vi "Set Combobox Font.vi"(6 "Combo Box Ref":refnum<vi>, 8 "error in (no error)":errorcluster, 9 "Font Size (0: No Change)":i32, 10 "Font (\"\": No Change)":string, 11 "Path Selector in":refnum<class "MGI Path Selector.lvclass">) -> (0 "error out":errorcluster, 3 "Path Selector out":refnum<class "MGI Path Selector.lvclass">)   [LabVIEW 2020, in "MGI Path Selector.lvclass"]
doc: "Update the specified combo box's font and size as specified.\n\nAuthored by Shawn Walpole\nsupport@mooregoodideas.com\nwww.mooregoodideas.com\n\nCopyright (c) 2013, Moore Good Ideas, Inc.\n\nAll rights reserved.\n\nRedistribution and use in source and binary forms, with or without modification, are permitted provided that the following conditions are met:\n\n * Redistributions of source code must retain the above copyright notice, this list of conditions and the following disclaimer.\n * Redistributions in binary form must reproduce the above copyright notice, this list of conditions and the following disclaimer in the documentation and/or other materials provided with the distribution.\n * Neither the name of Moore Good Ideas, Inc. nor the names of its contributors may be used to endorse or promote products derived from this software without specific prior written permission.\n\nTHIS SOFTWARE IS PROVIDED BY THE COPYRIGHT HOLDERS AND CONTRIBUTORS \"AS IS\" AND ANY EXPRESS OR IMPLIED WARRANTIES, INCLUDING, BUT NOT LIMITED TO, THE IMPLIED WARRANTIES OF MERCHANTABILITY AND FITNESS FOR A PARTICULAR PURPOSE ARE DISCLAIMED. IN NO EVENT SHALL THE COPYRIGHT OWNER OR CONTRIBUTORS BE LIABLE FOR ANY DIRECT, INDIRECT, INCIDENTAL, SPECIAL, EXEMPLARY, OR CONSEQUENTIAL DAMAGES (INCLUDING, BUT NOT LIMITED TO, PROCUREMENT OF SUBSTITUTE GOODS OR SERVICES; LOSS OF USE, DATA, OR PROFITS; OR BUSINESS INTERRUPTION) HOWEVER CAUSED AND ON ANY THEORY OF LIABILITY, WHETHER IN CONTRACT, STRICT LIABILITY, OR TORT (INCLUDING NEGLIGENCE OR OTHERWISE) ARISING IN ANY WAY OUT OF THE USE OF THIS SOFTWARE, EVEN IF ADVISED OF THE POSSIBILITY OF SUCH DAMAGE."
uses:
  <userlib>/_MGI/User Interface/Path Selector XControl/Class Hierarchy/MGI Path Selector.lvclass
  <userlib>/_MGI/User Interface/Path Selector XControl/Class Hierarchy/MGI Path Selector.lvclass/MGI Path Selector.ctl
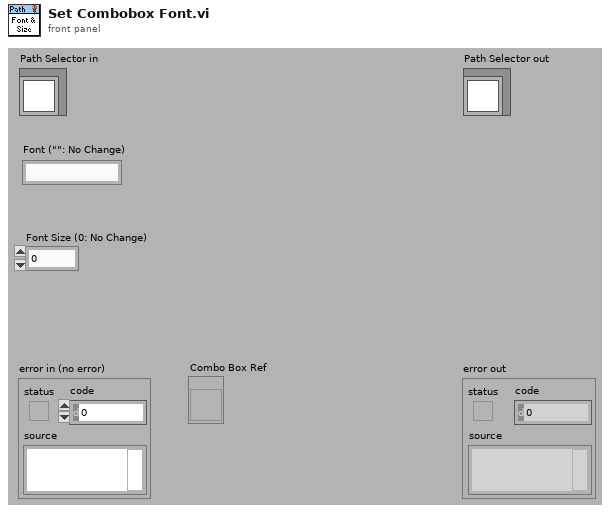
[diagram p1: front panel]
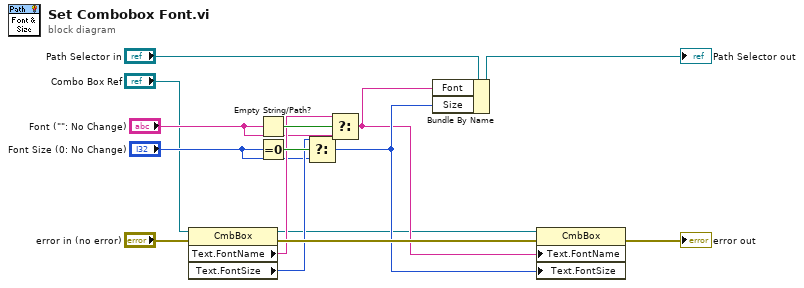
[diagram p0: block diagram]
diagram:
  n1 = property class="CmbBox"(reference="Combo Box Ref", error in="error in (no error)") -> (reference out=w1:refnum<vi>, error out=w9:errorcluster, "Text.FontName"=w8:string, "Text.FontSize"=w7:u32)
  n2 = Empty String/Path?(string/path="Font (\"\": No Change)") -> (empty?=w12:bool)
  n3 = Equal To 0?(x="Font Size (0: No Change)") -> (x = 0?=w11:bool)
  n4 = Select(t=w7, s=w11, f="Font Size (0: No Change)") -> (s? t:f=w4:u32)
  n5 = Select(t=w8, s=w12, f="Font (\"\": No Change)") -> (s? t:f=w3:string)
  n6 = Bundle By Name(cluster="Path Selector in", "Font"=w3, "Size"=w4) -> (→"Path Selector out":refnum<class "MGI Path Selector.lvclass">)
  n7 = property class="CmbBox"(reference=w1, error in=w9, "Text.FontName"=w3, "Text.FontSize"=w4) -> (error out=→"error out":errorcluster)  [unwired: 1 out]
